vi "Create Sysdef Tree Labels.vi"(6 "first call":bool, 7 "Autocreate Rx timestamp chans?":bool, 8 "error in":errorcluster, 9 "Labels":T2[](array[typedef]) {"scheduleBuildUnit" items=["Millisecond", "Microsecond"]}, 10 "Section Ptr":T1 format="%.0x", 11 "direction":T6) -> (0 "error out":errorcluster)   [LabVIEW 2016, in "Ballard Arinc-429 System Explorer.lvlib"]
uses:
  Ballard Arinc-429 System Explorer.lvlib
  <vilib>/NI Veristand/Custom Device API/Custom Device Channel Type.ctl
  <vilib>/NI Veristand/Custom Device API/Custom Device API.lvlib
  <vilib>/NI Veristand/Custom Device API/Custom Device Channel.ctl
  Shared/Controls and Global/Global.vi
  Shared/Ballard Arinc-429 Shared.lvlib
  Controls/Ballard_Label.ctl
  <vilib>/NI Veristand/Custom Device API/Custom Device Item Ref.ctl
  Controls/ARINCParam.ctl
  Controls/Ballard_Word.ctl
  Shared/Controls and Global/TransferType.ctl
  Controls/Channel_direction.ctl
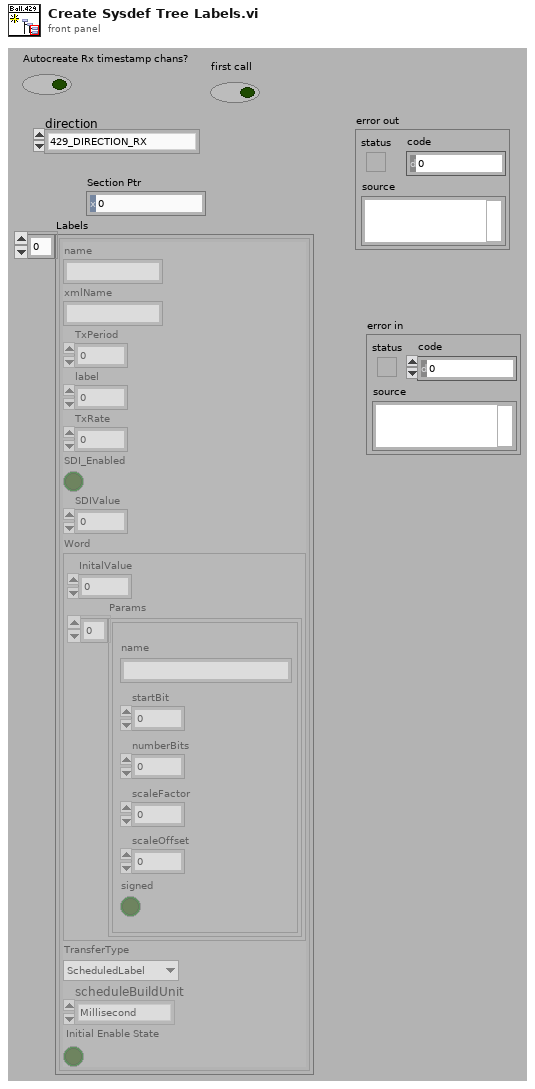
[diagram p1: front panel]
types:
  T1 = typedef "Custom Device API.lvlib/Custom Device Item Ref.ctl" = u64
  T2 = typedef "Ballard Arinc-429 System Explorer.lvlib/Ballard_Label.ctl" = cluster{"name":string, "xmlName":string, "TxPeriod":u32, "label":u32, "TxRate":dbl, "SDI_Enabled":bool, "SDIValue":u8, "Word":T3, "TransferType":T5, "scheduleBuildUnit":i32, "Initial Enable State":bool}
  T3 = typedef "Ballard Arinc-429 System Explorer.lvlib/Ballard_Word.ctl" = cluster{"InitalValue":u32, "Params":T4[]}
  T4 = typedef "Ballard Arinc-429 System Explorer.lvlib/ARINCParam.ctl" = cluster{"name":string, "startBit":i32, "numberBits":i32, "scaleFactor":dbl, "scaleOffset":dbl, "signed":bool}
  T5 = typedef "Ballard Arinc-429 Shared.lvlib/TransferType.ctl" = enum16{"ScheduledLabel", "Acyclic", "Block", "Strobe"}
  T6 = typedef "Ballard Arinc-429 System Explorer.lvlib/Channel_direction.ctl" = enum16{"429_DIRECTION_RX", "429_DIRECTION_TX"}
  T7 = typedef "Custom Device API.lvlib/Custom Device Channel.ctl" = cluster{"Type":T8, "Units":string, "Default Value":dbl, "Faultable":bool, "Scalable":bool}
  T8 = typedef "Custom Device API.lvlib/Custom Device Channel Type.ctl" = enum16{"Input", "Output"}
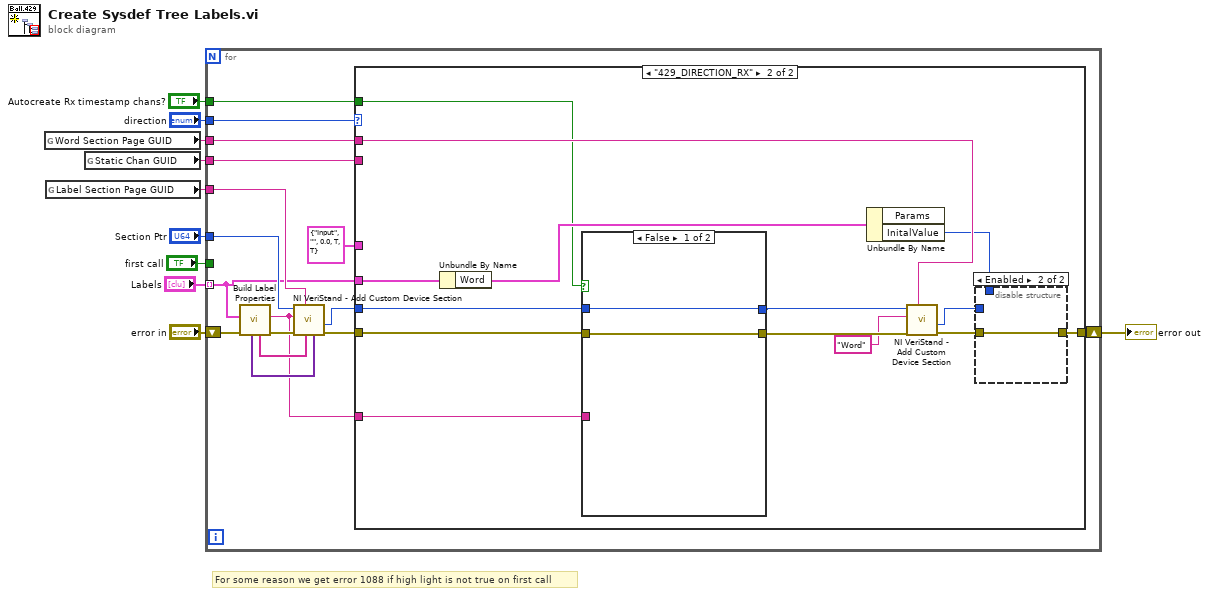
[diagram p0: block diagram]
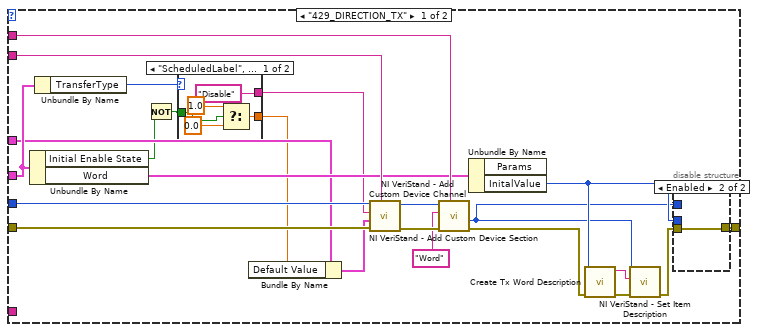
[diagram p2: hidden frame]
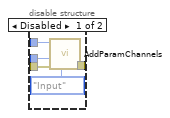
[diagram p3: hidden frame]
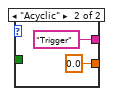
[diagram p4: hidden frame]
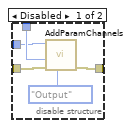
[diagram p5: hidden frame]
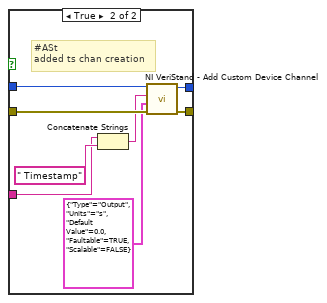
[diagram p6: hidden frame]
diagram:
  # "For some reason we get error 1088 if high light is not true on first call"
  n1 = global read "Global.vi" "Word Section Page GUID"() -> (w5:string)
  n2 = global read "Global.vi" "Label Section Page GUID"() -> (w7:string)
  n3 = global read "Global.vi" "Static Chan GUID"() -> (w6:string)
  n4 = for {
    shift-right: [w23] -> w4
    shift-left: "error in" -> [w15]
    tunnel: "Section Ptr" -> [w25]
    tunnel: "Labels" -> [w17] mode=indexing
    tunnel: "direction" -> [w22]
    tunnel: w7 -> [w20]
    tunnel: w6 -> [w19]
    tunnel: w5 -> [w16]
    tunnel: "first call" -> [_]
    tunnel: "Autocreate Rx timestamp chans?" -> [w12]
    n5 = call "Build Label Properties.vi"("error in (no error)"=w15, "Labels"=w17) -> ("error out"=w14:errorcluster, "name"=w11:string, "Prop Names"=w24:string[], "Prop Values"=w26:variant[])  [unwired: 6 in]
    n6 = call <vilib>:"NI VeriStand - Add Custom Device Section.vi"("Property Values"=w26, "Property names"=w24, "GUID (Default Section)"=w20, "error in (no error)"=w14, "Section Name"=w11, "Parent Ref in"=w25) -> ("error out"=w13:errorcluster, "Section Ptr"=w18:T1)  [unwired: 2 in, 2 out]
    n7 = case shown="\"429_DIRECTION_RX\"" w22 {
      tunnel: w13 -> [w47 w76]
      tunnel: w18 -> [w46 w73]
      tunnel: [w49 w75] -> w23
      tunnel: T7 {"Type"=enum."Input", "Units"="", "Default Value"=0.0, "Faultable"=TRUE, "Scalable"=TRUE} ("Channel") -> [w31 _]
      tunnel: w19 -> [w48 _]
      tunnel: w17 -> [w43 w74]
      tunnel: w16 -> [w45 w72]
      tunnel: w12 -> [_ w70]
      tunnel: w11 -> [_ w69]
      frame "429_DIRECTION_TX" {
        n8 = Unbundle By Name(w43) -> ("Initial Enable State"=w29:bool, "Word"=w44:T3)
        n9 = Unbundle By Name(w43) -> ("TransferType"=w42:T5)
        n10 = Not(x=w29) -> (.not. x?=w27:bool)
        n11 = case shown="\"ScheduledLabel\", Default" w42 {
          tunnel: ["Disable" ("Channel Name") "Trigger" ("Static Chan GUID")] -> w41
          tunnel: w27 -> [w57 _]
          tunnel: [w59 0.0] -> w28
          frame "ScheduledLabel", Default {
            n12 = Select(t=1.0, s=w57, f=0.0) -> (s? t:f=w59:dbl)
          }
          frame "Acyclic" {
          }
        }
        n13 = Bundle By Name(cluster=w31, "Default Value"=w28) -> (w30:T7)
        n14 = call <vilib>:"NI VeriStand - Add Custom Device Channel.vi"("GUID (Default Channel)"=w48, "error in (no error)"=w47, "Channel"=w30, "Channel Name"=w41, "Parent Ref in"=w46) -> ("error out"=w39:errorcluster, "Parent Ref out"=w40:T1)  [unwired: 3 in, 2 out]
        n15 = call <vilib>:"NI VeriStand - Add Custom Device Section.vi"("GUID (Default Section)"=w45, "error in (no error)"=w39, "Section Name"="Word" ("string"), "Parent Ref in"=w40) -> ("error out"=w38:errorcluster, "Section Ptr"=w34:T1)  [unwired: 4 in, 2 out]
        n16 = Unbundle By Name(w44) -> ("InitalValue"=w37:u32)  [unwired: 1 out]
        n17 = call "Create Tx Word Description.vi"("error in (no error)"=w38, "Initial Value"=w37) -> ("error out"=w36:errorcluster, "Description"=w35:string)  [unwired: 8 in]
        n18 = call <vilib>:"NI VeriStand - Set Item Description.vi"("error in (no error)"=w36, "Description"=w35, "Item Ref in"=w34) -> ("error out"=w33:errorcluster)  [unwired: 6 in, 2 out]
        n19 = disable-structure shown="Enabled" {
          disable-tunnel: [w54 w55] -> w49
          disable-tunnel: w37 -> [w52 _]
          disable-tunnel: w34 -> [w51 _]
          disable-tunnel: w33 -> [w50 w55]
          frame Disabled {
            n20 = call "AddParamChannels.vi"(6:Custom_Device_Channel_Type."Input" ("Type"), "error in"=w50, "HardwareChannel"=w52, "Node Ref In"=w51) -> ("error out"=w54:errorcluster)  [unwired: 6 in, 1 out]
          }
          frame Enabled {
          }
        }
      }
      frame "429_DIRECTION_RX" {
        n21 = Unbundle By Name(w74) -> ("Word"=w71:T3)
        n22 = case shown="False" w70 {
          tunnel: w76 -> [w84 w92]
          tunnel: [w84 w89] -> w65
          tunnel: w69 -> [_ w87]
          tunnel: w73 -> [w83 w86]
          tunnel: [w83 w85] -> w64
          frame False {
          }
          frame True {
            # "#ASt\nadded ts chan creation"
            n23 = Concatenate Strings(w87, " Timestamp" ("string")) -> (w91:string)
            n24 = call <vilib>:"NI VeriStand - Add Custom Device Channel.vi"("error in (no error)"=w92, "Channel"=T7 {"Type"=enum."Output", "Units"="s", "Default Value"=0.0, "Faultable"=TRUE, "Scalable"=FALSE}, "Channel Name"=w91, "Parent Ref in"=w86) -> ("error out"=w89:errorcluster, "Parent Ref out"=w85:T1)  [unwired: 4 in, 2 out]
          }
        }
        n25 = Unbundle By Name(w71) -> ("InitalValue"=w68:u32)  [unwired: 1 out]
        n26 = call <vilib>:"NI VeriStand - Add Custom Device Section.vi"("GUID (Default Section)"=w72, "error in (no error)"=w65, "Section Name"="Word" ("string"), "Parent Ref in"=w64) -> ("error out"=w67:errorcluster, "Section Ptr"=w66:T1)  [unwired: 4 in, 2 out]
        n27 = disable-structure shown="Enabled" {
          disable-tunnel: [w81 w82] -> w75
          disable-tunnel: w68 -> [w80 _]
          disable-tunnel: w67 -> [w79 w82]
          disable-tunnel: w66 -> [w77 _]
          frame Disabled {
            n28 = call "AddParamChannels.vi"(6:Custom_Device_Channel_Type."Output" ("Type"), "error in"=w79, "HardwareChannel"=w80, "Node Ref In"=w77) -> ("error out"=w81:errorcluster)  [unwired: 6 in, 1 out]
          }
          frame Enabled {
          }
        }
      }
    }
  }
  "error out" <- w4
